vi "TS_CloseReferences.vi"(0 "TestStand UI ExecutionView Manager":refnum<k7>, 1 "TabCtl Refnum":refnum<vi>, 2 "Str Refnum":refnum<vi>, 5 "TestStand UI SequenceFileView Manager":refnum<k7>, 7 "TestStand UI Application Manager (in)":refnum<k7>, 9 "Engine Ref in":refnum<k7>, 11 "error in":errorcluster) -> (10 "Shutdown":bool, 15 "error out":errorcluster)   [LabVIEW 2010]
uses:
  UI_Pages.ctl
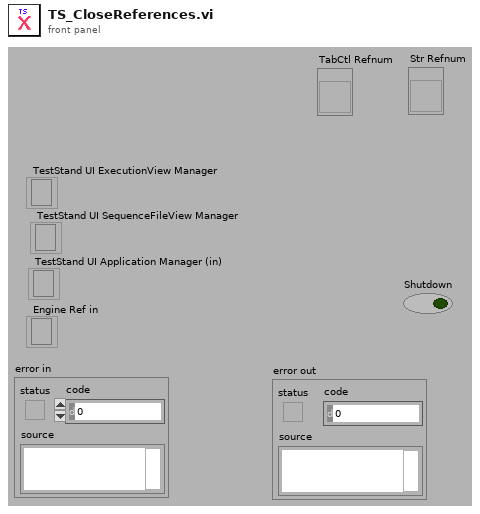
[diagram p1: front panel]
types:
  T1 = typedef "UI_Pages.ctl" = enum32{"Splash", "Test Script Builder", "Sequence Builder", "Report", "Utilities", "System Config"}
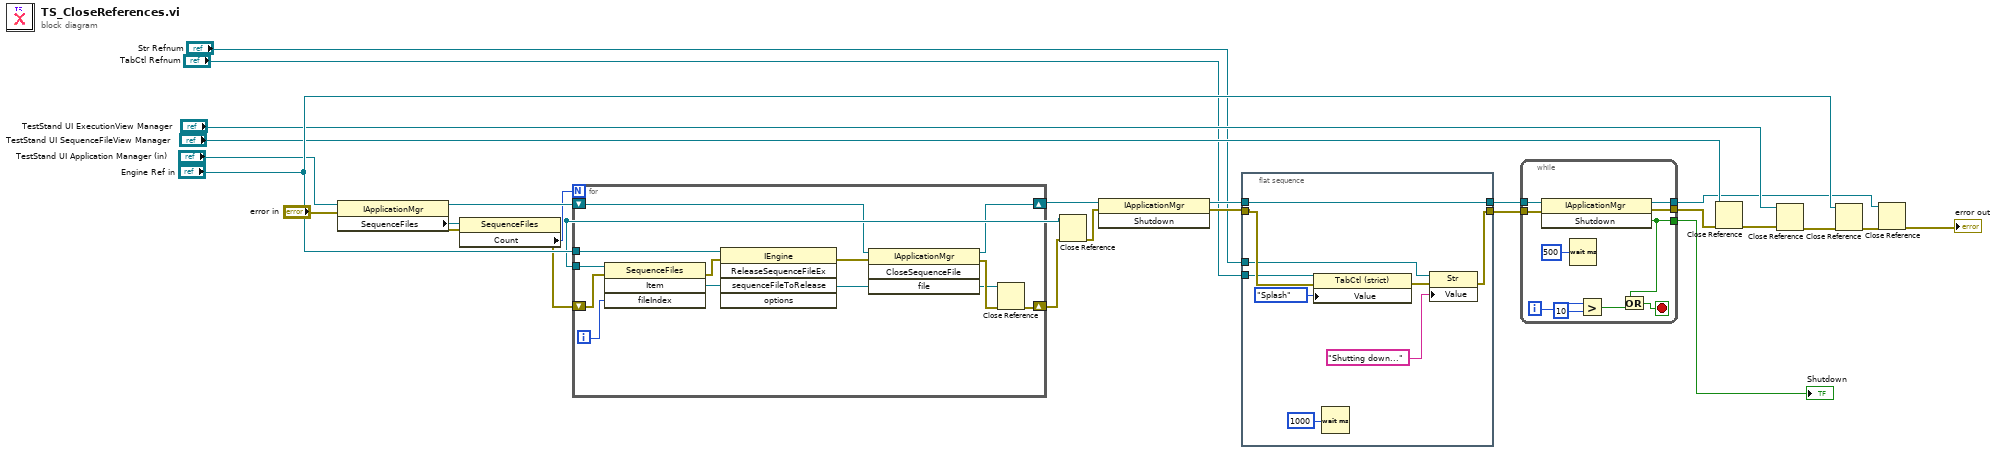
[diagram p0: block diagram]
diagram:
  n1 = property class="IApplicationMgr"(reference="TestStand UI Application Manager (in)", error in="error in") -> (reference out=w25:refnum<k7>, error out=w20:errorcluster, "SequenceFiles"=w17:refnum<k7>)
  n2 = property class="SequenceFiles"(reference=w17, error in=w20) -> (reference out=w1:refnum<k7>, error out=w21:errorcluster, "Count"=w18:i32)
  n3 = for {
    N: w18 -> [_]
    tunnel: "Engine Ref in" -> [w38]
    tunnel: w1 -> [w37]
    shift-right: [w28] -> w4
    shift-left: w25 -> [w34]
    shift-right: [w31] -> w3
    shift-left: w21 -> [w35]
    i -> [w36]
    n4 = invoke class="SequenceFiles" method="Item"(reference=w37, error in=w35, "fileIndex"=w36) -> (error out=w30:errorcluster, "Item"=w29:refnum<k7>)  [unwired: 1 in, 2 out]
    n5 = invoke class="IEngine" method="ReleaseSequenceFileEx"(reference=w38, error in=w30, "sequenceFileToRelease"=w29) -> (error out=w33:errorcluster)  [unwired: 2 in, 4 out]
    n6 = invoke class="IApplicationMgr" method="CloseSequenceFile"(reference=w34, error in=w33, "file"=w29) -> (reference out=w28:refnum<k7>, error out=w32:errorcluster)  [unwired: 1 in, 2 out]
    n7 = Close Reference(reference=w29, error in (no error)=w32) -> (error out=w31:errorcluster)
  }
  n8 = Close Reference(reference=w1, error in (no error)=w3) -> (error out=w2:errorcluster)
  n9 = invoke class="IApplicationMgr" method="Shutdown"(reference=w4, error in=w2) -> (reference out=w26:refnum<k7>, error out=w27:errorcluster)  [unwired: 1 in, 1 out]
  n10 = flat-sequence {
    tunnel: [w39] -> w10
    tunnel: [w44] -> w11
    tunnel: w27 -> [w45]
    tunnel: w26 -> [w44]
    tunnel: "TabCtl Refnum" -> [w42]
    tunnel: "Str Refnum" -> [w41]
    frame #0 {
      n11 = property on="Property Node" class="TabCtl (strict)"(reference=w42, error in=w45, "Value"=UI_Pages."Splash" ("State")) -> (error out=w40:errorcluster)  [unwired: 1 out]
      n12 = Wait (ms)(milliseconds to wait=u32 1000) -> ()  [unwired: 1 out]
      n13 = property on="Property Node" class="Str"(reference=w41, error in=w40, "Value"="Shutting down..." ("State")) -> (error out=w39:errorcluster)  [unwired: 1 out]
    }
  }
  n14 = while {
    tunnel: [w57] -> w15
    tunnel: [w48] -> w12
    tunnel: w11 -> [w56]
    tunnel: w10 -> [w55]
    tunnel: [w54] -> w9
    i -> [w50]
    stop <- w52 stop-if-true
    n15 = invoke class="IApplicationMgr" method="Shutdown"(reference=w56, error in=w55) -> (reference out=w57:refnum<k7>, error out=w54:errorcluster, "Shutdown"=w48:bool)  [unwired: 1 in]
    n16 = Wait (ms)(milliseconds to wait=u32 500) -> ()  [unwired: 1 out]
    n17 = Greater?(x=w50, y=10) -> (0:w51:bool)
    n18 = Or(x=w48, y=w51) -> (x .or. y?=w52:bool)
  }
  "Shutdown" <- w12
  n19 = Close Reference(reference="TestStand UI SequenceFileView Manager", error in (no error)=w9) -> (error out=w7:errorcluster)
  n20 = Close Reference(reference="TestStand UI ExecutionView Manager", error in (no error)=w7) -> (error out=w8:errorcluster)
  n21 = Close Reference(reference="Engine Ref in", error in (no error)=w8) -> (error out=w13:errorcluster)
  n22 = Close Reference(reference=w15, error in (no error)=w13) -> (error out=→"error out":errorcluster)
